vi "LEBITplc.CheckMon.vi"(0 "index of element":i32, 3 "i attribute in":T1, 5 "error in":errorcluster) -> (19 "error IO":errorcluster)   [LabVIEW 2014, in "LEBITplc.lvlib"]
uses:
  LEBITplc.lvlib
  LEBITplc.i attribute.ctl
panel:
  out "monValuePLC":string
  out "Monvalue":dbl
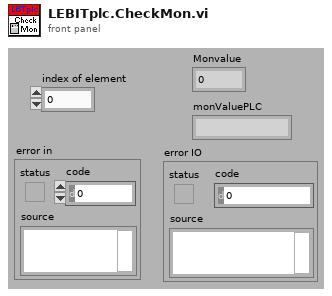
[diagram p1: front panel]
types:
  T1 = typedef "LEBITplc.lvlib/LEBITplc.i attribute.ctl" = cluster{"LLFLocation":string, "SetFileLocation":string, "nickNames":string[], "setValuePLCServiceID":i32[], "GUIServiceID":i32[], "monValuePLC":string[], "SetValueServiceID":i32[], "MonValueServiceID":i32[], "SetValue":dbl[][], "SetValueMin":dbl[], "SetValueMax":dbl[], "SetValueInfoServiceID":i32[], "GUINames":string[], "ListOfBases":string[], "Scale":dbl[], "Offset":dbl[], "setValuePLC":string[], "BaseName":string[], "ScaleServiceID":i32[], "OffsetServiceID":i32[], "AllPLCValues":string[], "CondSpecialArray":string[][], "CondSpecialIndex":i32[], "CondSpecialMonValue":dbl[], "RecentlyChanged":i32[], "SetFileLocationID":i32, "Dependent-Monitors":string[][], "LastLoadedFiles":string[], "IonGuideCalibLocation":string, "Monitor Dependent":string[], "Special":string[], "PLC?":bool[], "Start Date":string, "ListOfBasesServiceID":i32, "SETRA VISA resource":refnum<visa-resource-name>}
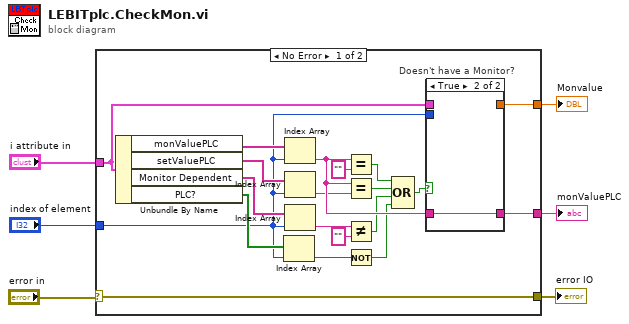
[diagram p0: block diagram]
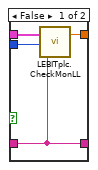
[diagram p2: hidden frame]
diagram:
  n1 = case shown="No Error" "error in" {
    selector: "error in" -> [w13 w32]
    tunnel: "i attribute in" -> [w16 _]
    tunnel: "index of element" -> [w9 _]
    tunnel: [w13 w32] -> w3
    tunnel: [w12 _] -> w2
    tunnel: [w11 _] -> w1
    frame No Error {
      n2 = Unbundle By Name(w16) -> ("monValuePLC"=w25:string[], "setValuePLC"=w24:string[], "Monitor Dependent"=w15:string[], "PLC?"=w10:bool[])
      n3 = Index Array(array=w10, index=w9) -> (element=w8:bool)
      n4 = Index Array(array=w25, index=w9) -> (element=w23:string)
      n5 = Index Array(array=w24, index=w9) -> (element=w22:string)
      n6 = Index Array(array=w15, index=w9) -> (element=w17:string)
      n7 = Equal?(x=w23, y="") -> (x = y?=w21:bool)
      n8 = Equal?(x=w23, y=w22) -> (x = y?=w20:bool)
      n9 = Not Equal?(x=w17, y="") -> (x != y?=w14:bool)
      n10 = Not(x=w8) -> (.not. x?=w7:bool)
      n11 = Compound Arithmetic op=OR(w21, w20, w14, w7) -> (w19:bool)
      n12 = case "Doesn't have a Monitor?" shown="True" w19 {
        tunnel: w23 -> [w29 w31]
        tunnel: [w29 w31] -> w11
        tunnel: [w30 _] -> w12
        tunnel: w16 -> [w28 _]
        tunnel: w9 -> [w27 _]
        frame False {
          n13 = call "LEBITplc.CheckMonLL.vi"("i attribute in"=w28, "index"=w27, "MonValuePLC"=w29) -> ("Monvalue"=w30:dbl)  [unwired: 16 in]
        }
        frame True {
        }
      }
    }
    frame Error {
    }
  }
  "error IO" <- w3
  "Monvalue" <- w2
  "monValuePLC" <- w1
